vi "Query Measurement Data Statistics.vi"(7 "Enable Recalculation (T: Enable)":bool=TRUE, 8 "error in (no error)":errorcluster, 9 "Reading Buffer (smua.nvbuffer1)":string="smua.nvbuffer1", 10 "Source Measure Unit Channel (0: Channel A)":i32(ring) items=["Channel A", "Channel B"], 11 "VISA resource name":refnum<visa-resource-name>) -> (0 "error out":errorcluster, 2 "Buffer Statistics":string[](array[string]), 3 "VISA resource name out":refnum<visa-resource-name>)   [LabVIEW 2017, in "Keithley 2600 Series.lvlib"]
doc: "Returns the statistical data about the data that is placed in the buffer."
uses:
  <instrlib>/Keithley 2600 Series/Keithley 2600 Series.lvlib
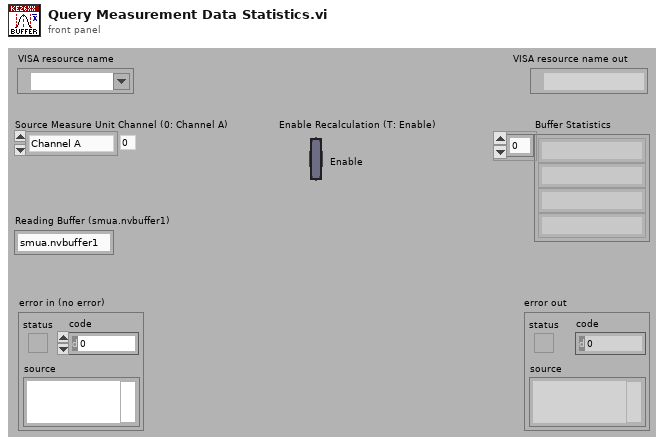
[diagram p1: front panel]
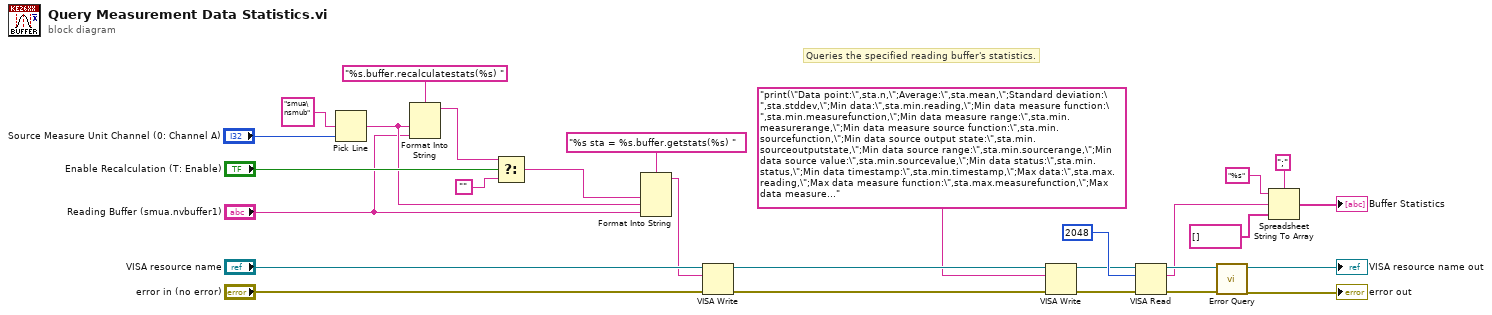
[diagram p0: block diagram]
diagram:
  # "Queries the specified reading buffer's statistics."
  n1 = Pick Line(multi-line string="smua\nsmub", line index="Source Measure Unit Channel (0: Channel A)") -> (output string=w16:string)  [unwired: 1 in]
  n2 = Format Into String(format string="%s.buffer.recalculatestats(%s) ", w16, "Reading Buffer (smua.nvbuffer1)") -> (resulting string=w19:string)  [unwired: 2 in, 1 out]
  n3 = Select(t=w19, s="Enable Recalculation (T: Enable)", f="") -> (s? t:f=w17:string)
  n4 = Format Into String(format string="%s sta = %s.buffer.getstats(%s) ", w17, w16, "Reading Buffer (smua.nvbuffer1)") -> (resulting string=w14:string)  [unwired: 2 in, 1 out]
  n5 = VISA Write(VISA resource name="VISA resource name", write buffer=w14, error in (no error)="error in (no error)") -> (VISA resource name out=w5:refnum<visa-resource-name>, error out=w3:errorcluster)  [unwired: 1 out]
  n6 = VISA Write(VISA resource name=w5, write buffer="print(\"Data point:\",sta.n,\";Average:\",sta.mean,\";Standard deviation:\",sta.stddev,\";Min data:\",sta.min.reading,\";Min data measure function:\",sta.min.measurefunction,\";Min data measure range:\",sta.min.measurerange,\";Min data measure source function:\",sta.min.sourcefunction,\";Min data source output state:\",sta.min.sourceoutputstate,\";Min data source range:\",sta.min.sourcerange,\";Min data source value:\",sta.min.sourcevalue,\";Min data status:\",sta.min.status,\";Min data timestamp:\",sta.min.timestamp,\";Max data:\",sta.max.reading,\";Max data measure function:\",sta.max.measurefunction,\";Max data measure range:\",sta.max.measurerange,\";Max data measure source function:\",sta.max.sourcefunction,\";Max data source output state:\",sta.max.sourceoutputstate,\";Max data source range:\",sta.max.sourcerange,\";Max data source value:\",sta.max.sourcevalue,\";Max data status:\",sta.max.status,\";Max data timestamp:\",sta.max.timestamp)", error in (no error)=w3) -> (VISA resource name out=w4:refnum<visa-resource-name>, error out=w2:errorcluster)  [unwired: 1 out]
  n7 = VISA Read(VISA resource name=w4, byte count=u32 2048, error in (no error)=w2) -> (VISA resource name out=w13:refnum<visa-resource-name>, read buffer=w10:string, error out=w12:errorcluster)  [unwired: 1 out]
  n8 = call <instrlib>:"Error Query.vi"("error in (no error)"=w12, "VISA resource name"=w13) -> ("error out"=→"error out":errorcluster, "VISA resource name out"=→"VISA resource name out":refnum<visa-resource-name>)  [unwired: 6 in, 2 out]
  n9 = Spreadsheet String To Array(delimiter (Tab)=";", format string="%s", spreadsheet string=w10, array type (2D Dbl)=string[] []) -> (array=→"Buffer Statistics":string[])
